vi "nonreentrant proc.vi"(8 "error in (no error)":errorcluster, 9 "parameters":T2, 10 "result allocation in":T2, 11 "Queue in":refnum<queue>) -> (0 "error out":errorcluster, 3 "result allocation out":T2)   [LabVIEW 2013, in "testmod runtime.lvclass"]
uses:
  testmod runtime.lvclass
  <vilib>/NI/Tag Bus/table/data table.ctl
  <vilib>/NI/Tag Bus Module Framework/runtime/error classification.ctl
  <vilib>/NI/Tag Bus Module Framework/runtime/TBM module execution interface.lvclass
  <vilib>/NI/Tag Bus/table/data table.lvlib
panel:
  in  "Numeric":dbl
  in  "error classification":T1=enum."none"
  in  "throw error":bool
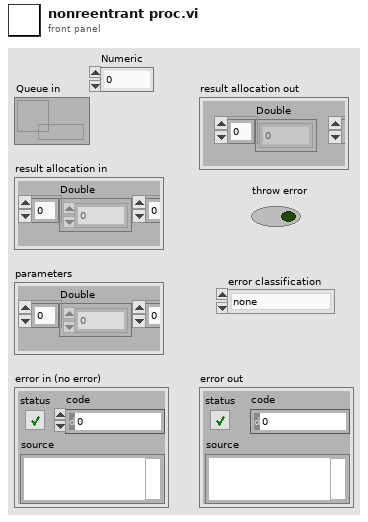
[diagram p1: front panel]
types:
  T1 = typedef "TBM module execution interface.lvclass/error classification.ctl" = enum16{"unknown", "none", "trivial", "recoverable", "critical"}
  T2 = typedef "tag bus.lvlib/data table.lvlib/data table.ctl" = cluster{"Double":dbl[], "Single":sgl[], "I64":i64[], "I32":i32[], "I16":i16[], "I8":i8[], "U64":u64[], "U32":u32[], "U16":u16[], "U8":u8[], "Boolean":bool[], "String":string[], "Array of Double":cluster{"DBL Array":dbl[]}[], "Array of Single":cluster{"SGL Array":sgl[]}[], "Array of I64":cluster{"I64 Array":i64[]}[], "Array of I32":cluster{"I32 Array":i32[]}[], "Array of I16":cluster{"I16 Array":i16[]}[], "Array of I8":cluster{"I8 Array":i8[]}[], "Array of U64":cluster{"U64 Array":u64[]}[], "Array of U32":cluster{"U32 Array":u32[]}[], "Array of U16":cluster{"U16 Array":u16[]}[], "Array of U8":cluster{"U8 Array":u8[]}[], "Array of Boolean":cluster{"Boolean Array":bool[]}[], "Array of String":cluster{"String Array":string[]}[]}
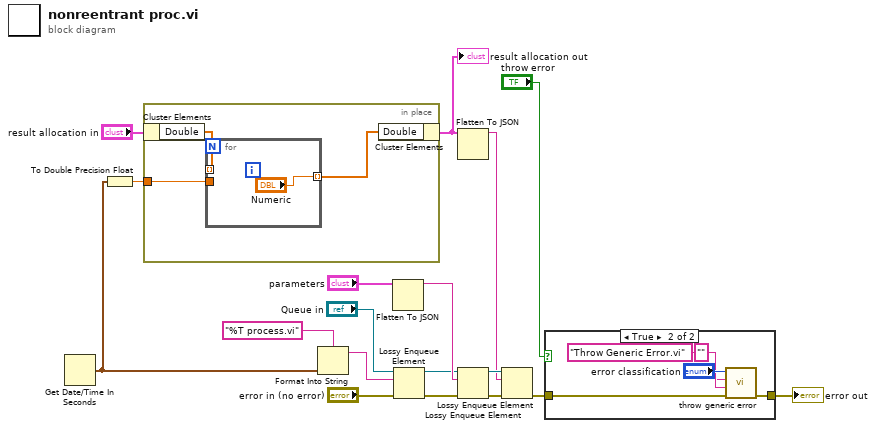
[diagram p0: block diagram]
diagram:
  n1 = Get Date/Time In Seconds() -> (seconds since 1Jan1904=w17:timestamp)
  n2 = To Double Precision Float(number=w17) -> (double precision float=w15:dbl)
  n3 = in-place {
    in-place-border: w15 -> [w20]
    n4 = in-place-cluster #1("result allocation in") -> ("Double"=w21:dbl[])
    n5 = for {
      tunnel: w21 -> [_] mode=indexing
      tunnel: w20 -> [_]
      tunnel: ["Numeric"] -> w19 mode=indexing
    }
    n6 = in-place-cluster #1("Double"=w19) -> (w7:T2)
  }
  "result allocation out" <- w7
  n7 = Format Into String(format string="%T process.vi", w17) -> (resulting string=w8:string)  [unwired: 2 in, 1 out]
  n8 = Flatten To JSON(anything="parameters") -> (JSON string=w13:string)  [unwired: 2 in, 1 out]
  n9 = Lossy Enqueue Element(queue="Queue in", element=w8, error in (no error)="error in (no error)") -> (queue out=w12:refnum<queue>, error out=w11:errorcluster)  [unwired: 2 out]
  n10 = Flatten To JSON(anything=w7) -> (JSON string=w4:string)  [unwired: 2 in, 1 out]
  n11 = Lossy Enqueue Element(queue=w12, element=w13, error in (no error)=w11) -> (queue out=w5:refnum<queue>, error out=w6:errorcluster)  [unwired: 2 out]
  n12 = Lossy Enqueue Element(queue=w5, element=w4, error in (no error)=w6) -> (error out=w3:errorcluster)  [unwired: 3 out]
  n13 = case shown="True" "throw error" {
    tunnel: w3 -> [w23 w28]
    tunnel: [w23 w27] -> w2
    frame False {
    }
    frame True {
      n14 = call <vilib>:"throw generic error.vi"("error in"=w28, "source"="Throw Generic Error.vi", "append error message"="", "error classification"="error classification") -> ("error out"=w27:errorcluster)  [unwired: 7 in]
    }
  }
  "error out" <- w2
